vi "global 2.vi"() -> ()   [LabVIEW 2015]
panel:
  in  "배열":u8[](array[numeric])
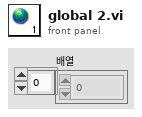
[diagram p1: front panel]
diagram:
